vi "FRIC_navX_Clear_Buffer_Warning.vi"(11 "error in":errorcluster) -> (3 "error out":errorcluster)   [LabVIEW 2016]
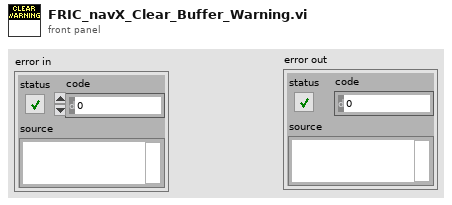
[diagram p1: front panel]
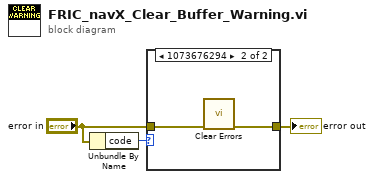
[diagram p0: block diagram]
diagram:
  n1 = Unbundle By Name("error in") -> ("code"=w2:i32)
  n2 = case shown="1073676294" w2 {
    tunnel: "error in" -> [w4 w6]
    tunnel: [w4 w5] -> w1
    frame 0, Default {
    }
    frame 1073676294 {
      n3 = call <vilib>:"Clear Errors.vi"("error in (no error)"=w6) -> ("error out"=w5:errorcluster)  [unwired: 5 in, 1 out]
    }
  }
  "error out" <- w1
